vi "HeartRate.vi"(8 "Remove Ectopic?":bool, 11 "Peaks X in":dbl[](array[numeric])) -> (1 "X [s]":dbl[](array[numeric]), 2 "RR intervals [ms]":dbl[](array[numeric]), 3 "Heart Rate [BPM]":dbl[](array[numeric]))   [LabVIEW 2014, in "Phonocardiography.lvlib"]
uses:
  Phonocardiography.lvlib
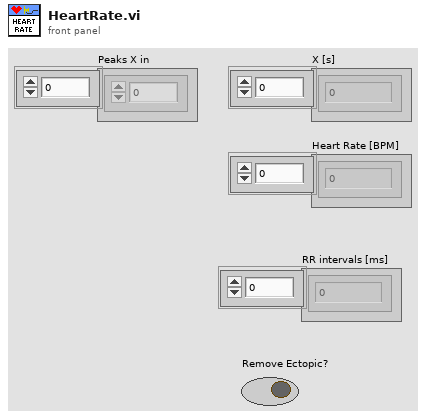
[diagram p1: front panel]
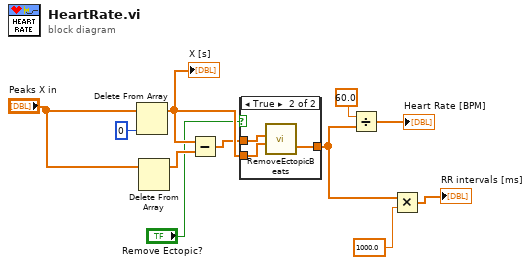
[diagram p0: block diagram]
diagram:
  n1 = Delete From Array(array="Peaks X in", index=0) -> (array with subset deleted=w5:dbl[])  [unwired: 1 in, 1 out]
  "X [s]" <- w5
  n2 = Delete From Array(array="Peaks X in") -> (array with subset deleted=w11:dbl[])  [unwired: 2 in, 1 out]
  n3 = Subtract(x=w5, y=w11) -> (x-y=w3:dbl[])
  n4 = case shown="True" "Remove Ectopic?" {
    tunnel: w5 -> [_ w15]
    tunnel: w3 -> [w12 w14]
    tunnel: [w12 w13] -> w2
    frame False {
    }
    frame True {
      n5 = call "RemoveEctopicBeats.vi"("X in [s]"=w15, "RR intervals in [s]"=w14) -> ("RR intervals out [s]"=w13:dbl[])  [unwired: 9 in]
    }
  }
  n6 = Divide(x=60.0, y=w2) -> (x/y=→"Heart Rate [BPM]":dbl[])
  n7 = Multiply(x=w2, y=1000.0) -> (x*y=→"RR intervals [ms]":dbl[])
